vi "StartPowerScan.vi"(0 "object in":refnum<class "InstrumentBase.lvclass">, 2 "PwrScanSettings":T1, 3 "CurrentProbeScaling(V/A)":dbl, 5 "error in (no error)":errorcluster) -> (14 "object out":refnum<class "InstrumentBase.lvclass">, 19 "error out":errorcluster)   [LabVIEW 2023, in "InstrumentBase.lvclass"]
uses:
  InstrumentBase.lvclass
  InstrumentBase.lvclass/InstrumentBase.ctl
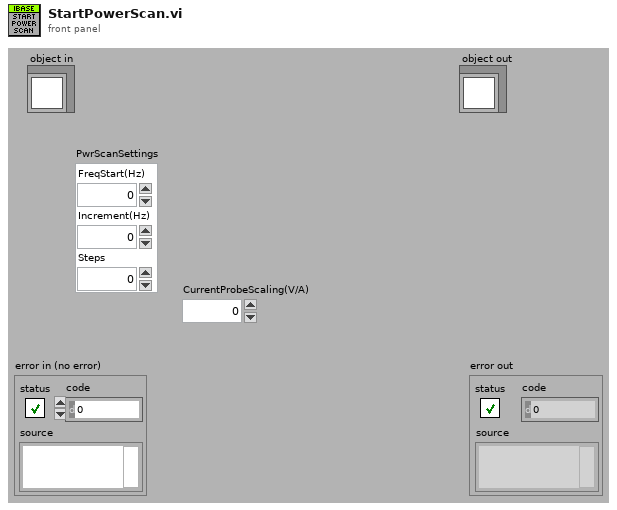
[diagram p1: front panel]
types:
  T1 = cluster{"FreqStart(Hz)":dbl, "Increment(Hz)":dbl, "Steps":i32}
  T2 = cluster{"Message":string, "Message Data":variant}
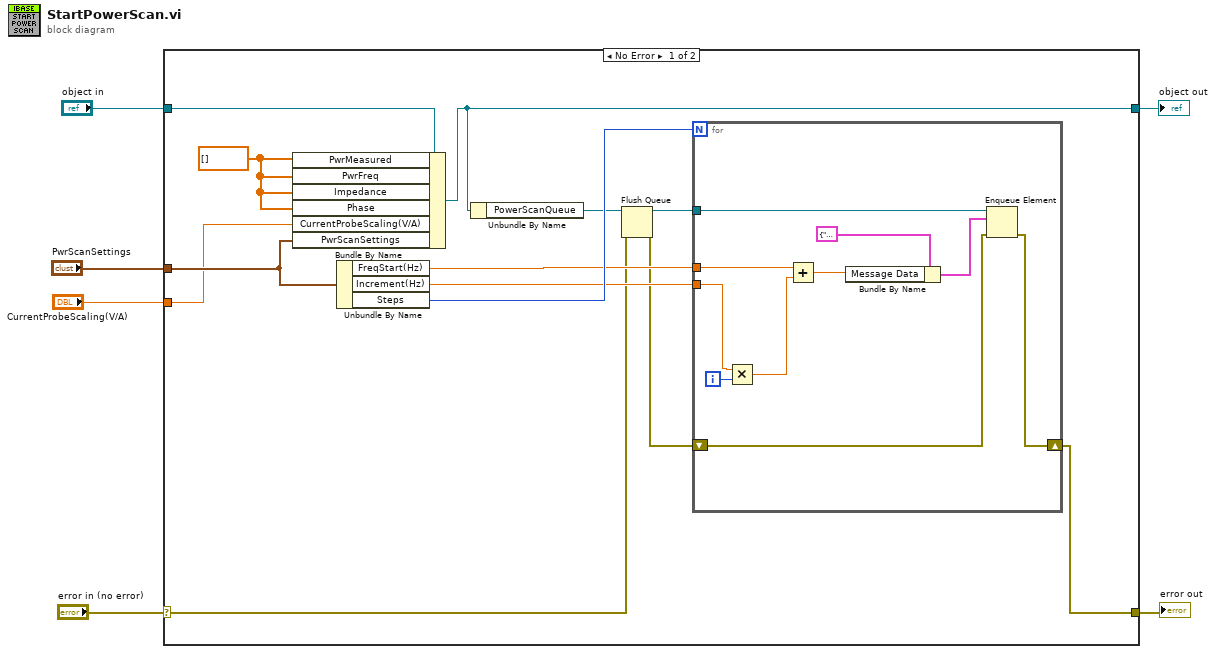
[diagram p0: block diagram]
diagram:
  n1 = case shown="No Error" "error in (no error)" {
    selector: "error in (no error)" -> [w11 w31]
    tunnel: [w14 w31] -> w5
    tunnel: [w18 w30] -> w3
    tunnel: "object in" -> [w19 w30]
    tunnel: "PwrScanSettings" -> [w9 _]
    tunnel: "CurrentProbeScaling(V/A)" -> [w8 _]
    frame No Error {
      w7 = dbl[] [] ("PwrMeasured")
      n2 = Bundle By Name(cluster=w19, "PwrMeasured"=w7, "PwrFreq"=w7, "Impedance"=w7, "Phase"=w7, "CurrentProbeScaling(V/A)"=w8, "PwrScanSettings"=w9) -> (w18:refnum<class "InstrumentBase.lvclass">)
      n3 = Unbundle By Name(w9) -> ("FreqStart(Hz)"=w16:dbl, "Increment(Hz)"=w15:dbl, "Steps"=w17:i32)
      n4 = Unbundle By Name(w18) -> ("PowerScanQueue"=w13:refnum<queue>)
      n5 = Flush Queue(queue=w13, error in (no error)=w11) -> (queue out=w12:refnum<queue>, error out=w10:errorcluster)  [unwired: 1 out]
      n6 = for {
        N: w17 -> [_]
        tunnel: w16 -> [w26]
        tunnel: w15 -> [w28]
        tunnel: w12 -> [w25]
        shift-right: [w21] -> w14
        shift-left: w10 -> [w20]
        i -> [w29]
        n7 = Multiply(x=w28, y=w29) -> (x*y=w27:dbl)
        n8 = Add(x=w26, y=w27) -> (x+y=w23:dbl)
        n9 = Bundle By Name(cluster=T2 {"Message"="", "Message Data"=variant} ("element"), "Message Data"=w23) -> (w22:T2)
        n10 = Enqueue Element(queue=w25, element=w22, error in (no error)=w20) -> (error out=w21:errorcluster)  [unwired: 1 in, 2 out]
      }
    }
    frame Error {
    }
  }
  "error out" <- w5
  "object out" <- w3
